vi "FindWindow.vi"(6 "error in (no error)":errorcluster, 9 "window name (\"\")":string) -> (0 "error out":errorcluster, 3 "hWnd":T1)   [LabVIEW 2011]
doc: "FindWindow\nThe FindWindow function retrieves a handle to the top-level window whose class name and window name match the specified strings. This function does not search child windows. This function does not perform a case-sensitive search. \n\nHWND FindWindow(\n LPCTSTR lpClassName, // pointer to class name\n LPCTSTR lpWindowName // pointer to window name\n);\n \nParameters\nlpClassName \nPointer to a null-terminated string that specifies the class name or is an atom that identifies the class-name string. If this parameter is an atom, it must be a global atom created by a previous call to theGlobalAddAtom function. The atom, a 16-bit value, must be placed in the low-order word of lpClassName; the high-order word must be zero. \nlpWindowName \nPointer to a null-terminated string that specifies the window name (the window's title). If this parameter is NULL, all window names match. \nReturn Values\nIf the function succeeds, the return value is a handle to the window that has the specified class name and window name.\n\nIf the function fails, the return value is NULL. To get extended error information, callGetLastError."
uses:
  hWnd.ctl
  user32.dll
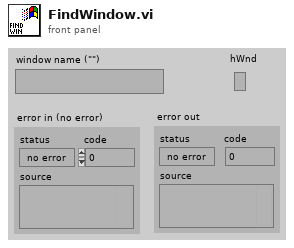
[diagram p1: front panel]
types:
  T1 = typedef "hWnd.ctl" = refnum<k1>
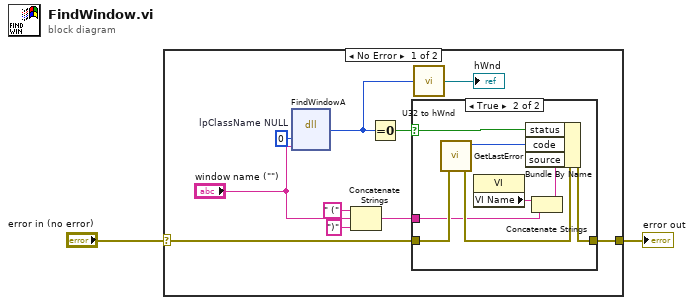
[diagram p0: block diagram]
diagram:
  n1 = case shown="No Error" "error in (no error)" {
    selector: "error in (no error)" -> [w10 w22]
    tunnel: [w12 w22] -> w2
    frame No Error {
      w7 = u32 0  # lpClassName NULL
      n2 = dll-call lib="user32.dll" fn="FindWindowA" label="FindWindow"("lpClassName"=w7, "lpWindowName"="window name (\"\")") -> ("hWnd"=w9:u32)  [unwired: 5 in, 2 out]
      n3 = Concatenate Strings(" (" ("string"), "window name (\"\")", ")" ("string")) -> (w6:string)
      n4 = Equal To 0?(x=w9) -> (x = 0?=w11:bool)
      n5 = case shown="True" w11 {
        selector: w11 -> [_ w20]
        tunnel: w10 -> [w13 w18]
        tunnel: [w13 w21] -> w12
        tunnel: w6 -> [_ w14]
        frame False {
        }
        frame True {
          n6 = call "GetLastError.vi"("error in (no error)"=w18) -> ("error out"=w17:errorcluster, "CODE"=w19:i32)  [unwired: 5 out]
          n7 = property class="VI"() -> ("VI Name"=w16:string)  [unwired: 2 in, 2 out]
          n8 = Concatenate Strings(w16, w14) -> (w15:string)
          n9 = Bundle By Name(cluster=w17, "status"=w20, "code"=w19, "source"=w15) -> (w21:errorcluster)
        }
      }
      n10 = call "U32 to hWnd.vi"("hWnd"=w9) -> ("hWnd"=→"hWnd":T1)  [unwired: 4 out]
    }
    frame Error {
    }
  }
  "error out" <- w2
